vi "Enable Disable FP.vi"(10 "Disabled":T1(ring)=enum."Disabled and Grayed Out", 11 "cluster":T2) -> (0 "error out":errorcluster)   [LabVIEW 2025]
doc: "Enable or disable the FP controls and indicators."
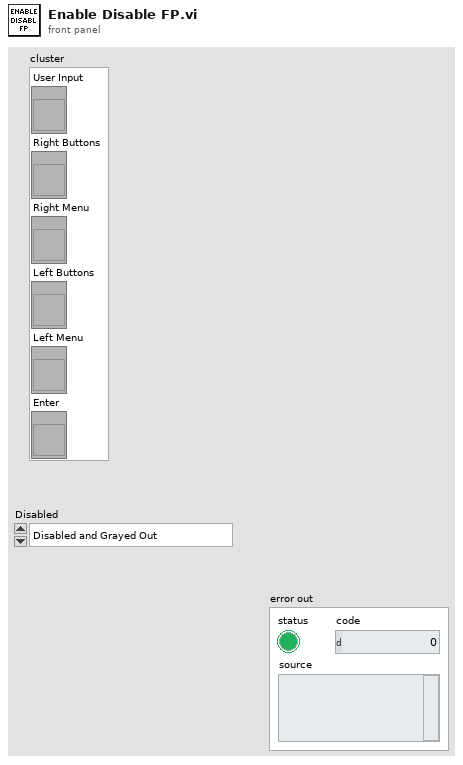
[diagram p1: front panel]
types:
  T1 = enum8{"Enabled", "Disabled", "Disabled and Grayed Out"}
  T2 = cluster{"User Input":refnum<vi>, "Right Buttons":refnum<vi>, "Right Menu":refnum<vi>, "Left Buttons":refnum<vi>, "Left Menu":refnum<vi>, "Enter":refnum<vi>}
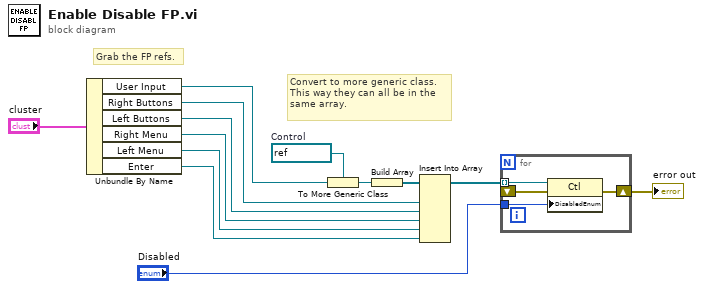
[diagram p0: block diagram]
diagram:
  w4 = refnum<vi> refnum  # Control
  # "Convert to more generic class.\nThis way they can all be in the\nsame array."
  # "Grab the FP refs."
  n1 = Unbundle By Name("cluster") -> ("User Input"=w9:refnum<vi>, "Right Buttons"=w10:refnum<vi>, "Left Buttons"=w6:refnum<vi>, "Right Menu"=w7:refnum<vi>, "Left Menu"=w8:refnum<vi>, "Enter"=w13:refnum<vi>)
  n2 = To More Generic Class(target class=w4, reference=w9) -> (generic class reference=w5:refnum<vi>)
  n3 = Build Array(w5) -> (w3:refnum<vi>[])
  n4 = Insert Into Array(array=w3, new element #1=w10, new element #2=w6, new element #3=w7, new element #4=w8, new element #5=w13) -> (w11:refnum<vi>[])  [unwired: 1 in]
  n5 = for {
    tunnel: w11 -> [w17] mode=indexing
    tunnel: "Disabled" -> [w16]
    shift-right: [w15] -> w1
    shift-left: _ -> [w14]
    n6 = property on="Property Node" class="Ctl"(reference=w17, error in=w14, "DisabledEnum"=w16) -> (error out=w15:errorcluster)  [unwired: 1 out]
  }
  "error out" <- w1
